vi "Send UpdtCamTestCntrlEvnts.vi"(7 "Message Priority (Normal)":T7=enum."Normal", 8 "error in (no error)":errorcluster, 10 "CameraTestingEvnt":T1, 11 "Message Enqueuer":refnum<class "Message Enqueuer.lvclass">) -> (0 "error out":errorcluster, 3 "Message Enqueuer out":refnum<class "Message Enqueuer.lvclass">)   [LabVIEW 2020, in "ICameraTestingUI.lvlib" / "UpdtCamTestCntrlEvnts Msg.lvclass"]
doc: "This VI sends the message to an actor."
uses:
  UpdtCamTestCntrlEvnts Msg.lvclass
  UpdtCamTestCntrlEvnts Msg.lvclass/UpdtCamTestCntrlEvnts Msg.ctl
  <vilib>/ActorFramework/Message Enqueuer/Message Enqueuer.lvclass
  C:/Program Files (x86)/National Instruments/LabVIEW 2020/vi.lib/ActorFramework/Message/Message.lvclass
  E:/GitHub/Evaluation_Test/Labview/src/CameraTestingApp/ICameraTestingUI/ICameraTestingUI Messages/UpdtCamTestCntrlEvnts Msg/UpdtCamTestCntrlEvnts Msg.lvclass
  <vilib>/ActorFramework/Message Enqueuer/Message Priority.ctl
  Camera/ICamera/ICamera/TypeDef/SnapInfo.ctl
  Camera/ICamera/ICamera/ICamera.lvclass
  ICameraTesting/ICameraTesting/TypeDef/FrameRateValReceived.ctl
  ICameraTesting/ICameraTesting/ICameraTesting.lvclass
  ICameraTesting/ICameraTesting/TypeDef/ImgTypeValReceived.ctl
  ICameraTesting/ICameraTesting/TypeDef/ResolutionValReceived.ctl
  Camera/ICamera/ICamera/TypeDef/VideoOptionsCodes.ctl
  ICameraTesting/ICameraTesting/TypeDef/VideoOptCodesReceived.ctl
  ICameraTesting/ICameraTesting/TypeDef/StatusLogUpdate.ctl
  ICameraTesting/ICameraTesting/TypeDef/Events.ctl
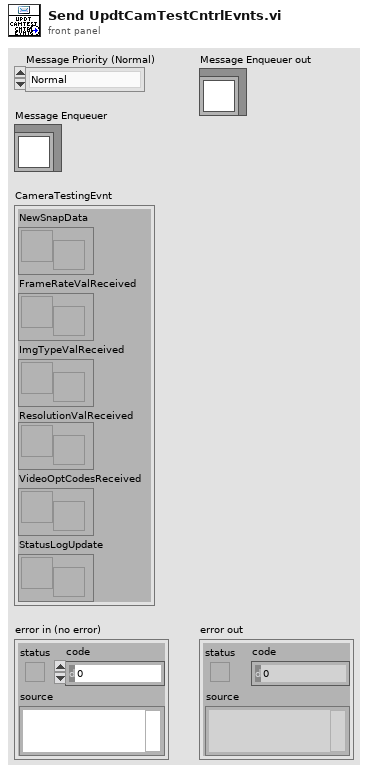
[diagram p1: front panel]
types:
  T1 = typedef "ICameraTesting.lvlib/ICameraTesting.lvclass/Events.ctl" = cluster{"NewSnapData":refnum<user-event>, "FrameRateValReceived":T2, "ImgTypeValReceived":T3, "ResolutionValReceived":T4, "VideoOptCodesReceived":T5, "StatusLogUpdate":T6}
  T2 = typedef "ICameraTesting.lvlib/ICameraTesting.lvclass/FrameRateValReceived.ctl" = refnum<user-event>
  T3 = typedef "ICameraTesting.lvlib/ICameraTesting.lvclass/ImgTypeValReceived.ctl" = refnum<user-event>
  T4 = typedef "ICameraTesting.lvlib/ICameraTesting.lvclass/ResolutionValReceived.ctl" = refnum<user-event>
  T5 = typedef "ICameraTesting.lvlib/ICameraTesting.lvclass/VideoOptCodesReceived.ctl" = refnum<user-event>
  T6 = typedef "ICameraTesting.lvlib/ICameraTesting.lvclass/StatusLogUpdate.ctl" = refnum<user-event>
  T7 = typedef "Actor Framework.lvlib/Message Enqueuer.lvclass/Message Priority.ctl" = enum16{"Low", "Normal", "High"}
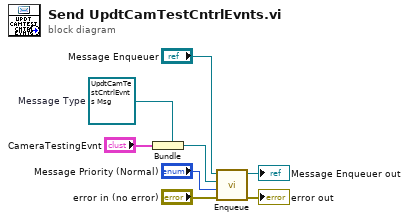
[diagram p0: block diagram]
diagram:
  w5 = refnum<class "UpdtCamTestCntrlEvnts Msg.lvclass"> refnum  # Message Type
  n1 = Bundle(cluster=w5, "CameraTestingEvnt") -> (w4:refnum<class "UpdtCamTestCntrlEvnts Msg.lvclass">)
  n2 = call <vilib>:"Enqueue.vi"("error in (no error)"="error in (no error)", "Message Priority (Normal)"="Message Priority (Normal)", "Message"=w4, "Message Enqueuer in"="Message Enqueuer") -> ("error out"=→"error out":errorcluster, "Message Enqueuer in"=→"Message Enqueuer out":refnum<class "Message Enqueuer.lvclass">)  [unwired: 6 in]
